vi "Test Boards_OBJECT.vi"() -> ()   [LabVIEW 2023]
doc: "See <b>Read_Me.html</b> in the <b>Board Testing</b> project for a detailed description of this VI."
uses:
  Common/Board Image.ctl
  Board/Board Design.lvclass
panel:
  out "Test Results":T2(array[cluster])
  # "Overview: Demonstrates an object-based solution to a board testing problem.\n\nSee Read_Me.html in the project for a detailed description of this VI."
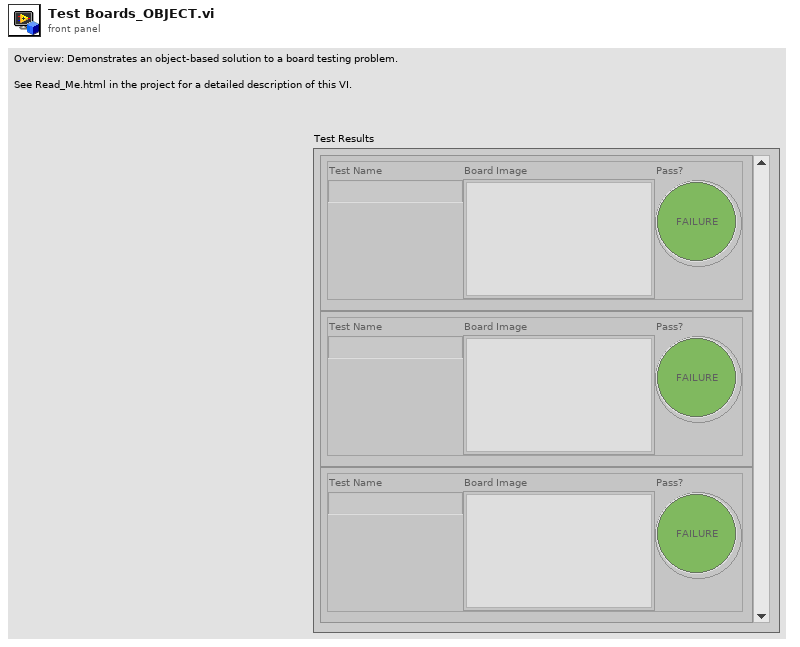
[diagram p1: front panel]
types:
  T1 = typedef "Board Image.ctl" = picture
  T2 = cluster{"Test Name":string, "Board Image":T1, "Pass?":bool}[]
  T3 = typedef "Assembly Line Input.ctl" = cluster{"board image":T1, "which board":T4}
  T4 = typedef "Board Type Enum.ctl" = enum16{"Basic DAQ Board", "Elite DAQ Board", "GPIB Board"}
  T5 = typedef "Pass Fail Boolean.ctl" = bool
  T6 = cluster{"test name":string, "board image":T1, "pass?":T5}
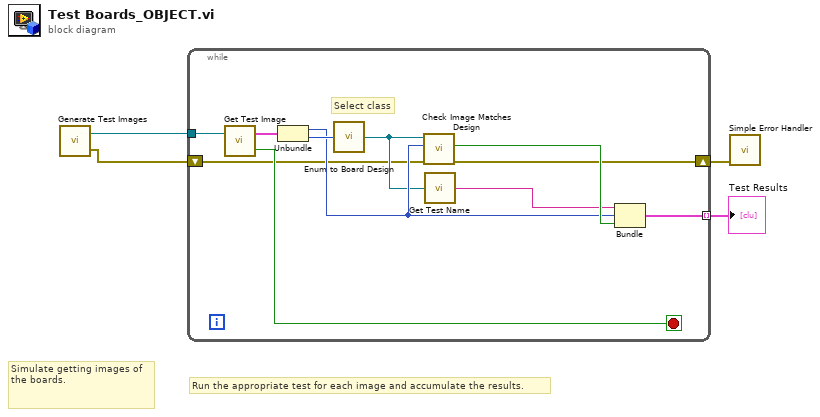
[diagram p0: block diagram]
diagram:
  # "Run the appropriate test for each image and accumulate the results."
  # "Simulate getting images of the boards."
  n1 = call "Generate Test Images.vi"() -> ("error out"=w2:errorcluster, "queue out"=w4:refnum<queue>)  [unwired: 2 in]
  n2 = while {
    tunnel: w4 -> [w14]
    tunnel: [w9] -> w3 mode=indexing
    shift-right: [w6] -> w1
    shift-left: w2 -> [w5]
    stop <- w13 stop-if-true
    # "Select class"
    n3 = call "Get Test Image.vi"("queue in"=w14) -> ("no more images after this?"=w13:bool, "Assembly Line Image"=w12:T3)  [unwired: 1 in]
    n4 = Unbundle(w12) -> ("board image"=w10:T1, "which board"=w11:T4)
    n5 = call "Enum to Board Design.vi"("which board"=w11) -> ("board.lvclass"=w7:refnum<class "Board Design.lvclass">)
    n6 = call-dynamic "Check Image Matches Design.vi"("error in"=w5, "board image"=w10, "board in"=w7) -> ("error out"=w6:errorcluster, "pass?"=w15:T5)  [unwired: 6 in, 1 out]
    n7 = call "Get Test Name.vi"("board in"=w7) -> ("test name"=w8:string)
    n8 = Bundle("test name"=w8, "board image"=w10, "pass?"=w15) -> (w9:T6)  [unwired: 1 in]
  }
  "Test Results" <- w3
  n9 = call <vilib>:"Simple Error Handler.vi"("error in (no error)"=w1) -> ()  [unwired: 4 in, 5 out]
